vi "EnabletChannelVI.vi"(0 "Angelsample":dbl[](array[numeric]), 1 "Angel":bool[](array[boolean]), 2 "dt":dbl, 5 "Torquesample":dbl[](array[numeric]), 7 "Torque":bool[](array[boolean]), 9 "ResetAngel":dbl[](array[numeric]), 11 "ResetTorqueCommand":dbl[](array[numeric]), 12 "ChannelSetArray":T1[](array[typedef]) {"Enable" items=["不使能", "使能"]; "Wave" items=["0指令", "正弦波", "方波", "三角波", "常值", "波形数据", "白噪声", "正弦扫频", "梯度加载", "VMIC"]; "ChannelType" items=["标准波形跟踪"=1, "扫频测试"=2, "消除多余力"=3, "梯度加载"=4, "载荷谱跟踪"=5, "模拟输入跟踪"=9]; "ChannelStatus" items=["通道关", "位置通道", "加载通道"]}, 13 "AxisForceSample":dbl[](array[numeric])) -> (4 "OutPut":dbl[](array[numeric]), 6 "resetAngel 2":dbl[](array[numeric]), 10 "ResetTorque 2":dbl[](array[numeric]), 15 "Commandout":dbl[](array[numeric]))   [LabVIEW 2014]
uses:
  ChannelCommand.ctl
  Control 1.ctl
  WaveType.ctl
  MoterEnable.ctl
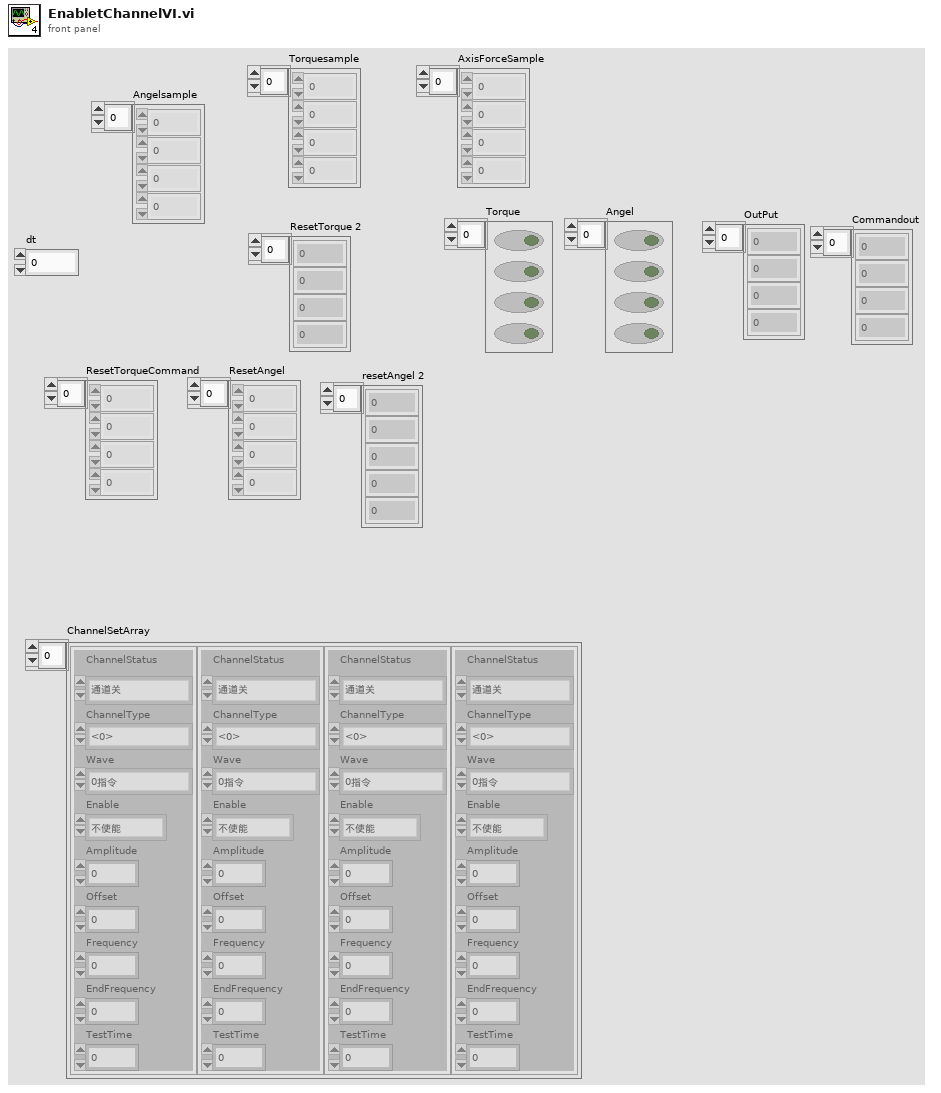
[diagram p1: front panel]
types:
  T1 = typedef "ChannelCommand.ctl" = cluster{"ChannelStatus":T2, "ChannelType":i32, "Wave":T3, "Enable":T4, "Amplitude":dbl, "Offset":dbl, "Frequency":dbl, "EndFrequency":dbl, "TestTime":dbl}
  T2 = typedef "Control 1.ctl" = i32
  T3 = typedef "WaveType.ctl" = i32
  T4 = typedef "MoterEnable.ctl" = u16
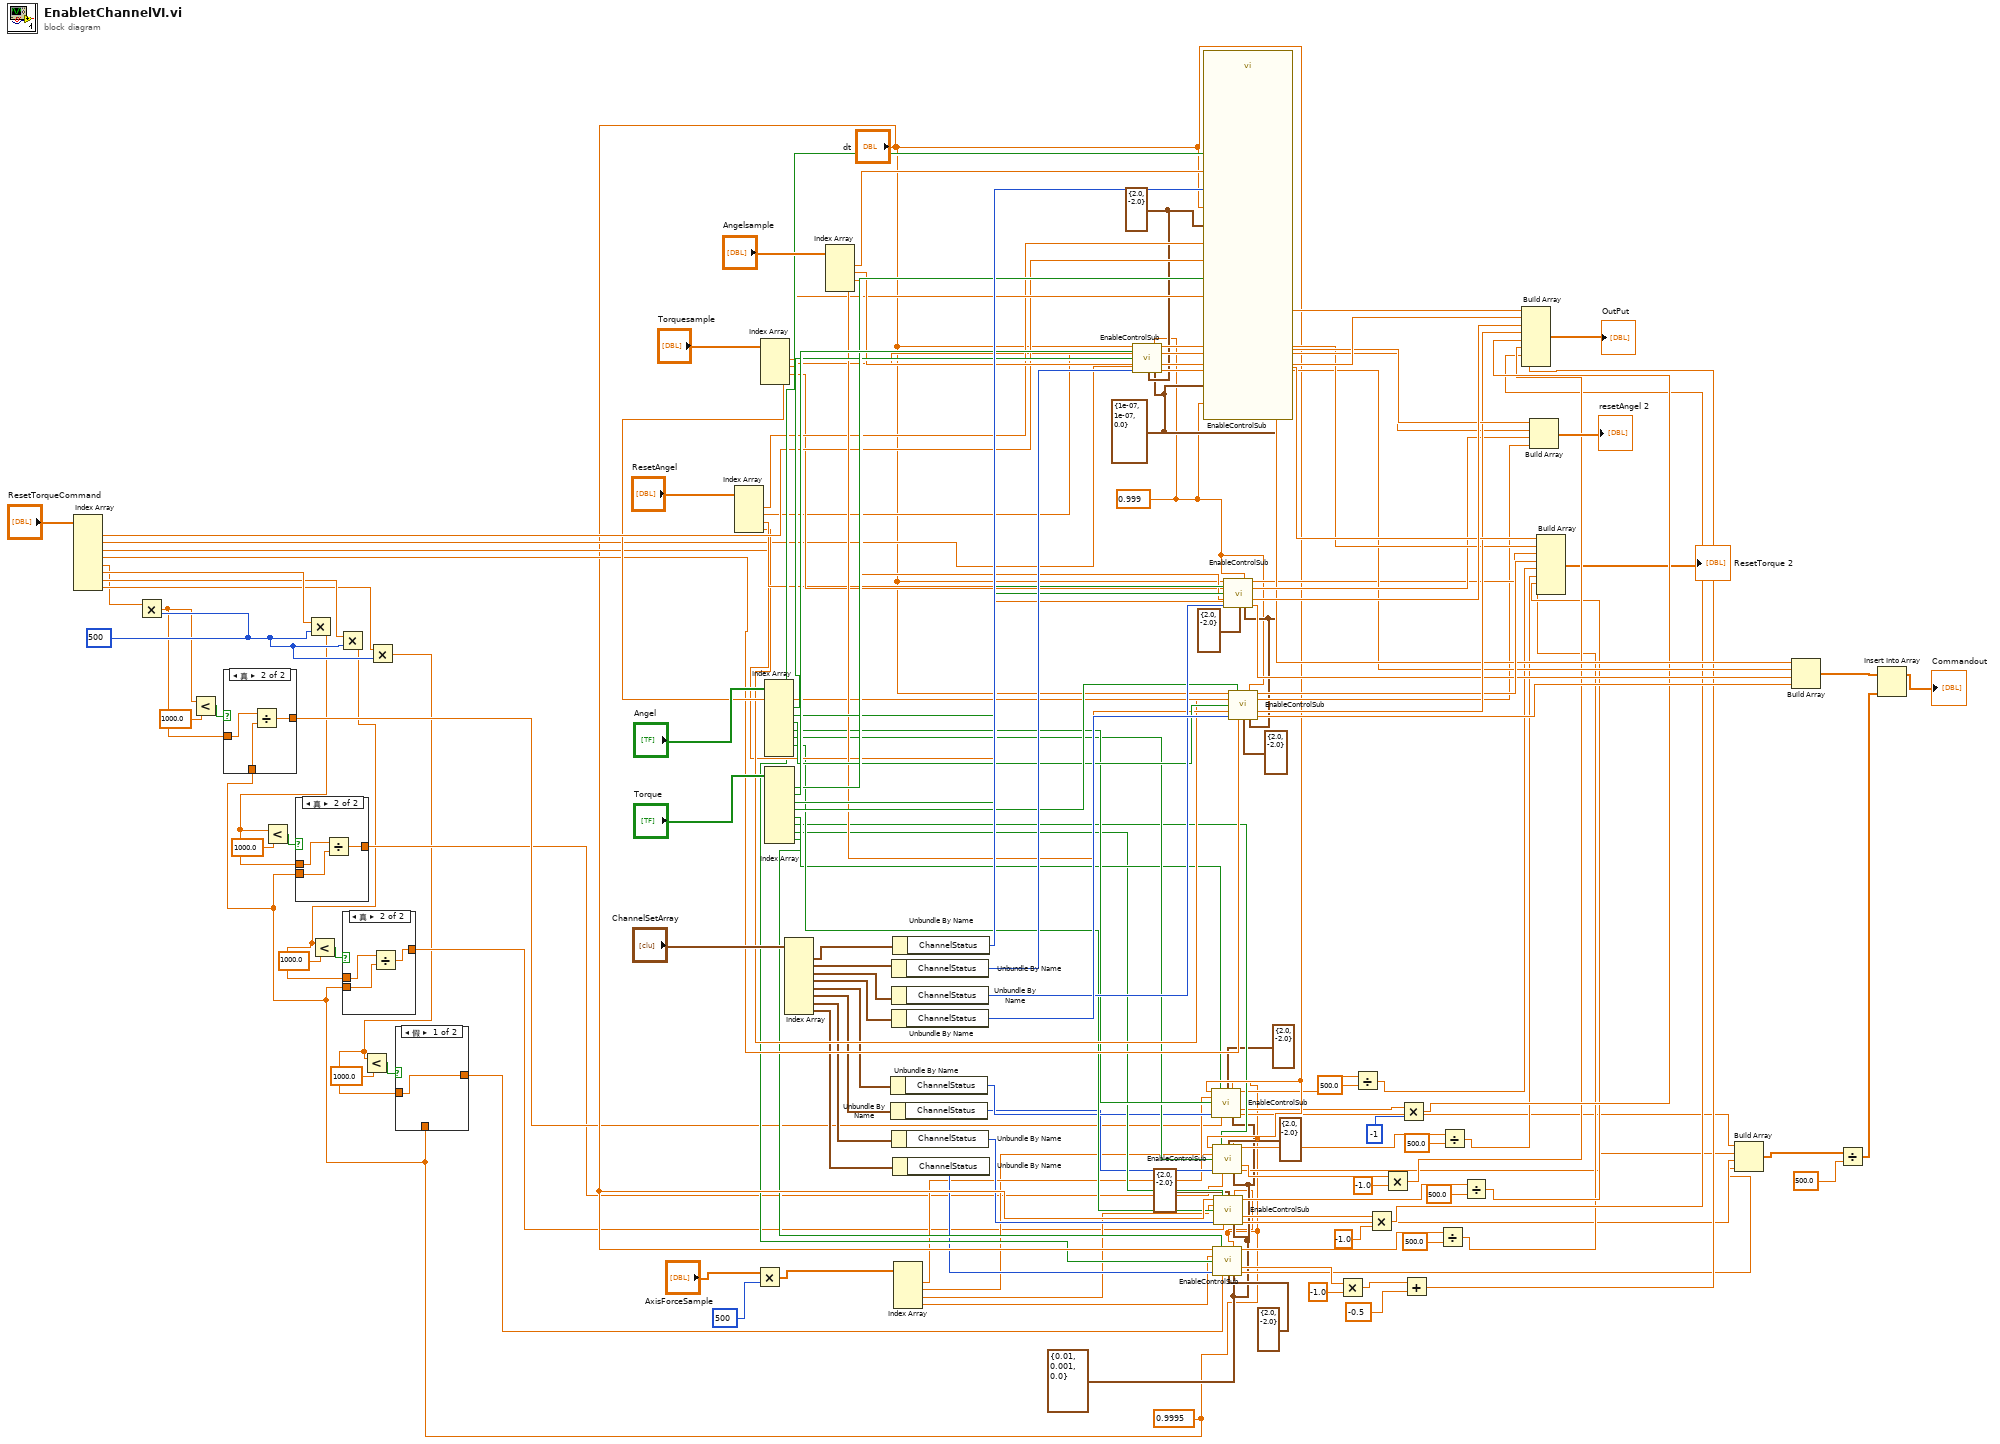
[diagram p0: block diagram]
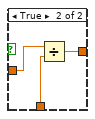
[diagram p2: hidden frame]
diagram:
  w1 = 0.9995
  w2 = 0.999
  w3 = cluster{dbl, dbl, dbl} {0.01, 0.001, 0.0} ("簇")
  w4 = cluster{dbl, dbl, dbl} {1e-07, 1e-07, 0.0} ("簇")
  w60 = 500
  w5 = cluster{"output high":dbl, "output low":dbl} {"output high"=2.0, "output low"=-2.0} ("output range")
  n1 = Index Array(array="ResetTorqueCommand") -> (element #1=w118:dbl, element #2=w111:dbl, element #3=w110:dbl, element #4=w109:dbl, element #5=w42:dbl, element #6=w63:dbl, element #7=w62:dbl, element #8=w61:dbl)  [unwired: 8 in]
  n2 = Multiply(x=w42, y=w60) -> (x*y=w41:dbl)
  n3 = Less?(x=w41, y=1000.0) -> (x < y?=w43:bool)
  n4 = case shown="真" w43 {
    tunnel: w41 -> [w150 w153]
    tunnel: [w150 w152] -> w40
    tunnel: w1 -> [_ w151]
    frame False {
    }
    frame True {
      n5 = Divide(x=w153, y=w151) -> (x/y=w152:dbl)
    }
  }
  n6 = Multiply(x=w63, y=w60) -> (x*y=w33:dbl)
  n7 = Less?(x=w33, y=1000.0) -> (x < y?=w38:bool)
  n8 = case shown="真" w38 {
    tunnel: w33 -> [w154 w157]
    tunnel: [w154 w156] -> w32
    tunnel: w1 -> [_ w155]
    frame False {
    }
    frame True {
      n9 = Divide(x=w157, y=w155) -> (x/y=w156:dbl)
    }
  }
  n10 = Multiply(x=w62, y=w60) -> (x*y=w31:dbl)
  n11 = Less?(x=w31, y=1000.0) -> (x < y?=w36:bool)
  n12 = case shown="真" w36 {
    tunnel: w31 -> [w158 w161]
    tunnel: [w158 w160] -> w30
    tunnel: w1 -> [_ w159]
    frame False {
    }
    frame True {
      n13 = Divide(x=w161, y=w159) -> (x/y=w160:dbl)
    }
  }
  n14 = Multiply(x=w61, y=w60) -> (x*y=w29:dbl)
  n15 = Less?(x=w29, y=1000.0) -> (x < y?=w34:bool)
  n16 = case shown="假" w34 {
    tunnel: w29 -> [w162 w165]
    tunnel: [w162 w164] -> w28
    tunnel: w1 -> [_ w163]
    frame False {
    }
    frame True {
      n17 = Divide(x=w165, y=w163) -> (x/y=w164:dbl)
    }
  }
  n18 = Index Array(array="ResetAngel") -> (element #1=w119:dbl, element #2=w114:dbl, element #3=w113:dbl, element #4=w112:dbl)  [unwired: 4 in]
  n19 = Multiply(x="AxisForceSample", y=500) -> (x*y=w57:dbl[])
  n20 = Index Array(array="Torquesample") -> (element #1=w120:dbl, element #2=w117:dbl, element #3=w116:dbl, element #4=w115:dbl)  [unwired: 4 in]
  n21 = Index Array(array="Angel") -> (element #1=w125:bool, element #2=w126:bool, element #3=w127:bool, element #4=w128:bool, element #5=w87:bool, element #6=w86:bool, element #7=w85:bool, element #8=w84:bool)  [unwired: 8 in]
  n22 = Index Array(array="Torque") -> (element #1=w129:bool, element #2=w130:bool, element #3=w131:bool, element #4=w132:bool, element #5=w83:bool, element #6=w82:bool, element #7=w81:bool, element #8=w80:bool)  [unwired: 8 in]
  n23 = Index Array(array="ChannelSetArray") -> (element #1=w142:T1, element #2=w141:T1, element #3=w140:T1, element #4=w139:T1, element #5=w92:T1, element #6=w91:T1, element #7=w90:T1, element #8=w89:T1)  [unwired: 8 in]
  n24 = Index Array(array="Angelsample") -> (element #1=w124:dbl, element #2=w123:dbl, element #3=w122:dbl, element #4=w121:dbl)  [unwired: 4 in]
  n25 = Unbundle By Name(w92) -> ("ChannelStatus"=w79:T2)
  n26 = Unbundle By Name(w91) -> ("ChannelStatus"=w78:T2)
  n27 = Unbundle By Name(w141) -> ("ChannelStatus"=w136:T2)
  n28 = Unbundle By Name(w140) -> ("ChannelStatus"=w137:T2)
  n29 = Unbundle By Name(w139) -> ("ChannelStatus"=w138:T2)
  n30 = Unbundle By Name(w90) -> ("ChannelStatus"=w77:T2)
  n31 = Unbundle By Name(w142) -> ("ChannelStatus"=w135:T2)
  n32 = Unbundle By Name(w89) -> ("ChannelStatus"=w76:T2)
  n33 = Index Array(array=w57) -> (element #1=w75:dbl, element #2=w72:dbl, element #3=w74:dbl, element #4=w73:dbl)  [unwired: 4 in]
  n34 = call "EnableControlSub.vi"("dt"="dt", "Torque"=w130, "ResetAngle"=w114, "复位速率"=w2, "TorqueSample0"=w117, "Angel"=w126, "AngleSample0"=w123, "ChannelStatus"=w136, "ResetTorque"=w111, "output range"=w5, "簇"=w4) -> ("ResetTorque 2"=w101:dbl, "ResetAngle 2"=w102:dbl, "ControlOutput"=w107:dbl, "Commandout"=w97:dbl)  [unwired: 1 in]
  n35 = call "EnableControlSub.vi"("dt"="dt", "Torque"=w129, "ResetAngle"=w119, "复位速率"=w2, "TorqueSample0"=w120, "Angel"=w125, "AngleSample0"=w124, "ChannelStatus"=w135, "ResetTorque"=w118, "output range"=w5, "簇"=w4) -> ("ResetTorque 2"=w104:dbl, "ResetAngle 2"=w105:dbl, "ControlOutput"=w108:dbl, "Commandout"=w98:dbl)  [unwired: 1 in]
  n36 = call "EnableControlSub.vi"("dt"="dt", "Torque"=w83, "复位速率"=w1, "TorqueSample0"=w75, "Angel"=w87, "ChannelStatus"=w79, "ResetTorque"=w40, "output range"=cluster{"output high":dbl, "output low":dbl} {"output high"=2.0, "output low"=-2.0}, "簇"=w3) -> ("ResetTorque 2"=w25:dbl, "ControlOutput"=w56:dbl, "Commandout"=w14:dbl)  [unwired: 3 in, 1 out]
  n37 = call "EnableControlSub.vi"("dt"="dt", "Torque"=w82, "复位速率"=w1, "TorqueSample0"=w72, "Angel"=w86, "ChannelStatus"=w78, "ResetTorque"=w32, "output range"=cluster{"output high":dbl, "output low":dbl} {"output high"=2.0, "output low"=-2.0}, "簇"=w3) -> ("ResetTorque 2"=w22:dbl, "ControlOutput"=w53:dbl, "Commandout"=w13:dbl)  [unwired: 3 in, 1 out]
  n38 = call "EnableControlSub.vi"("dt"="dt", "Torque"=w80, "复位速率"=w1, "TorqueSample0"=w73, "Angel"=w84, "ChannelStatus"=w76, "ResetTorque"=w28, "output range"=cluster{"output high":dbl, "output low":dbl} {"output high"=2.0, "output low"=-2.0}, "簇"=w3) -> ("ResetTorque 2"=w16:dbl, "ControlOutput"=w47:dbl, "Commandout"=w11:dbl)  [unwired: 3 in, 1 out]
  n39 = call "EnableControlSub.vi"("dt"="dt", "Torque"=w81, "复位速率"=w1, "TorqueSample0"=w74, "Angel"=w85, "ChannelStatus"=w77, "ResetTorque"=w30, "output range"=cluster{"output high":dbl, "output low":dbl} {"output high"=2.0, "output low"=-2.0}, "簇"=w3) -> ("ResetTorque 2"=w19:dbl, "ControlOutput"=w50:dbl, "Commandout"=w12:dbl)  [unwired: 3 in, 1 out]
  n40 = call "EnableControlSub.vi"("dt"="dt", "Torque"=w131, "ResetAngle"=w113, "复位速率"=w2, "TorqueSample0"=w116, "Angel"=w127, "AngleSample0"=w122, "ChannelStatus"=w137, "ResetTorque"=w110, "output range"=cluster{"output high":dbl, "output low":dbl} {"output high"=2.0, "output low"=-2.0}, "簇"=w4) -> ("ResetTorque 2"=w94:dbl, "ResetAngle 2"=w100:dbl, "ControlOutput"=w106:dbl, "Commandout"=w96:dbl)  [unwired: 1 in]
  n41 = call "EnableControlSub.vi"("dt"="dt", "Torque"=w132, "ResetAngle"=w112, "复位速率"=w2, "TorqueSample0"=w115, "Angel"=w128, "AngleSample0"=w121, "ChannelStatus"=w138, "ResetTorque"=w109, "output range"=cluster{"output high":dbl, "output low":dbl} {"output high"=2.0, "output low"=-2.0}, "簇"=w4) -> ("ResetTorque 2"=w99:dbl, "ResetAngle 2"=w93:dbl, "ControlOutput"=w103:dbl, "Commandout"=w95:dbl)  [unwired: 1 in]
  n42 = Multiply(x=w47, y=-1.0) -> (x*y=w46:dbl)
  n43 = Divide(x=w25, y=500.0) -> (x/y=w24:dbl)
  n44 = Multiply(x=w50, y=-1.0) -> (x*y=w49:dbl)
  n45 = Multiply(x=w53, y=-1.0) -> (x*y=w52:dbl)
  n46 = Multiply(x=w56, y=-1) -> (x*y=w54:dbl)
  n47 = Add(x=w46, y=-0.5) -> (x+y=w65:dbl)
  n48 = Divide(x=w16, y=500.0) -> (x/y=w15:dbl)
  n49 = Divide(x=w22, y=500.0) -> (x/y=w21:dbl)
  n50 = Divide(x=w19, y=500.0) -> (x/y=w18:dbl)
  n51 = Build Array(w108, w107, w106, w103, w54, w52, w49, w65) -> (→"OutPut":dbl[])
  n52 = Build Array(w105, w102, w100, w93) -> (→"resetAngel 2":dbl[])
  n53 = Build Array(w104, w101, w94, w99, w24, w21, w18, w15) -> (→"ResetTorque 2":dbl[])
  n54 = Build Array(w14, w13, w12, w11) -> (w9:dbl[])
  n55 = Build Array(w98, w97, w96, w95) -> (w7:dbl[])
  n56 = Divide(x=w9, y=500.0) -> (x/y=w8:dbl[])
  n57 = Insert Into Array(array=w7, new element=w8) -> (→"Commandout":dbl[])  [unwired: 1 in]
